vi "Check for Connection Request.vi"(8 "error in (no error)":errorcluster, 9 "timeout ms (25000)":i32, 11 "connection ID in":refnum<k5>) -> (0 "error out":errorcluster, 1 "timed out?":bool, 2 "buffer descriptor":T1, 3 "connection ID out":refnum<k5>)   [LabVIEW 2017, in "DSF Core.lvlib" / "Data Server Thread.lvclass"]
uses:
  Data Server Thread.lvclass
  Buffer Descriptor.ctl
  Buffer Type.ctl
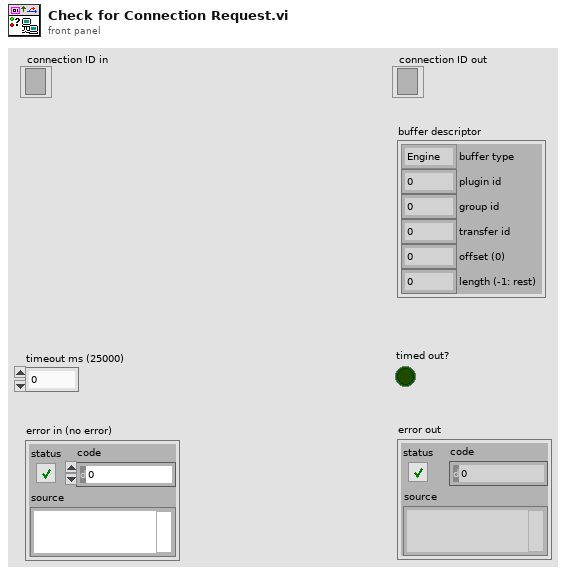
[diagram p1: front panel]
types:
  T1 = typedef "DSF Core.lvlib/Data Server Thread.lvclass/Buffer Descriptor.ctl" = cluster{"buffer type":T2, "plugin id":i32, "group id":i32, "transfer id":i32, "offset (0)":u64, "length (-1: rest)":i64}
  T2 = typedef "DSF Core.lvlib/Data Server Thread.lvclass/Buffer Type.ctl" = enum16{"Engine", "String"}
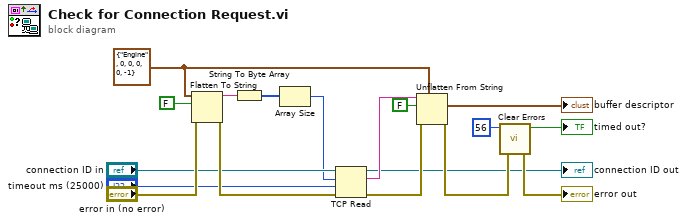
[diagram p0: block diagram]
diagram:
  w9 = T1 {"buffer type"=enum."Engine", "plugin id"=0, "group id"=0, "transfer id"=0, "offset (0)"=0, "length (-1: rest)"=-1} ("Cluster")
  n1 = Flatten To String(anything=w9, prepend array or string size? (T)=FALSE, error in (no error)="error in (no error)") -> (data string=w15:string, error out=w16:errorcluster)  [unwired: 1 in, 1 out]
  n2 = String To Byte Array(string=w15) -> (unsigned byte array=w14:u8[])
  n3 = Array Size(array=w14) -> (size(s)=w12:i32)
  n4 = TCP Read(connection ID="connection ID in", bytes to read=w12, error in (no error)=w16, 9:"timeout ms (25000)") -> (connection ID out=→"connection ID out":refnum<k5>, data out=w10:string, error out=w11:errorcluster)  [unwired: 1 in]
  n5 = Unflatten From String(type=w9, binary string=w10, data includes array or string size? (T)=FALSE, error in (no error)=w11) -> (value=→"buffer descriptor":T1, error out=w5:errorcluster)  [unwired: 1 in, 1 out]
  n6 = call <vilib>:"Clear Errors.vi"("error in (no error)"=w5, "specific error code to clear (0: all)"=56) -> ("error out"=→"error out":errorcluster, "specific error cleared?"=→"timed out?":bool)  [unwired: 4 in]
